vi "Remove Digital Pattern.vi"(8 "error in (no error)":errorcluster, 10 "Page Data in":T1 {"Node Ptr" format="%.0x"}, 11 "State queue in":string[](array[string])) -> (0 "error out":errorcluster, 2 "Page Data out":T1 {"Node Ptr" format="%.0x"}, 3 "State queue out":string[](array[string]))   [LabVIEW 2013, in "Engine Simulation Toolkit System Explorer.lvlib"]
uses:
  Engine Simulation Toolkit System Explorer.lvlib
  Digital Patterns Page Data.ctl
  <vilib>/NI Veristand/Custom Device API/Custom Device Item Ref.ctl
  Digital Pattern.ctl
  Digital Pattern Base.ctl
  Digital Pattern Remove Edge.ctl
  Digital Pattern Add Pulse.ctl
  <vilib>/NI Veristand/Custom Device API/Custom Device API.lvlib
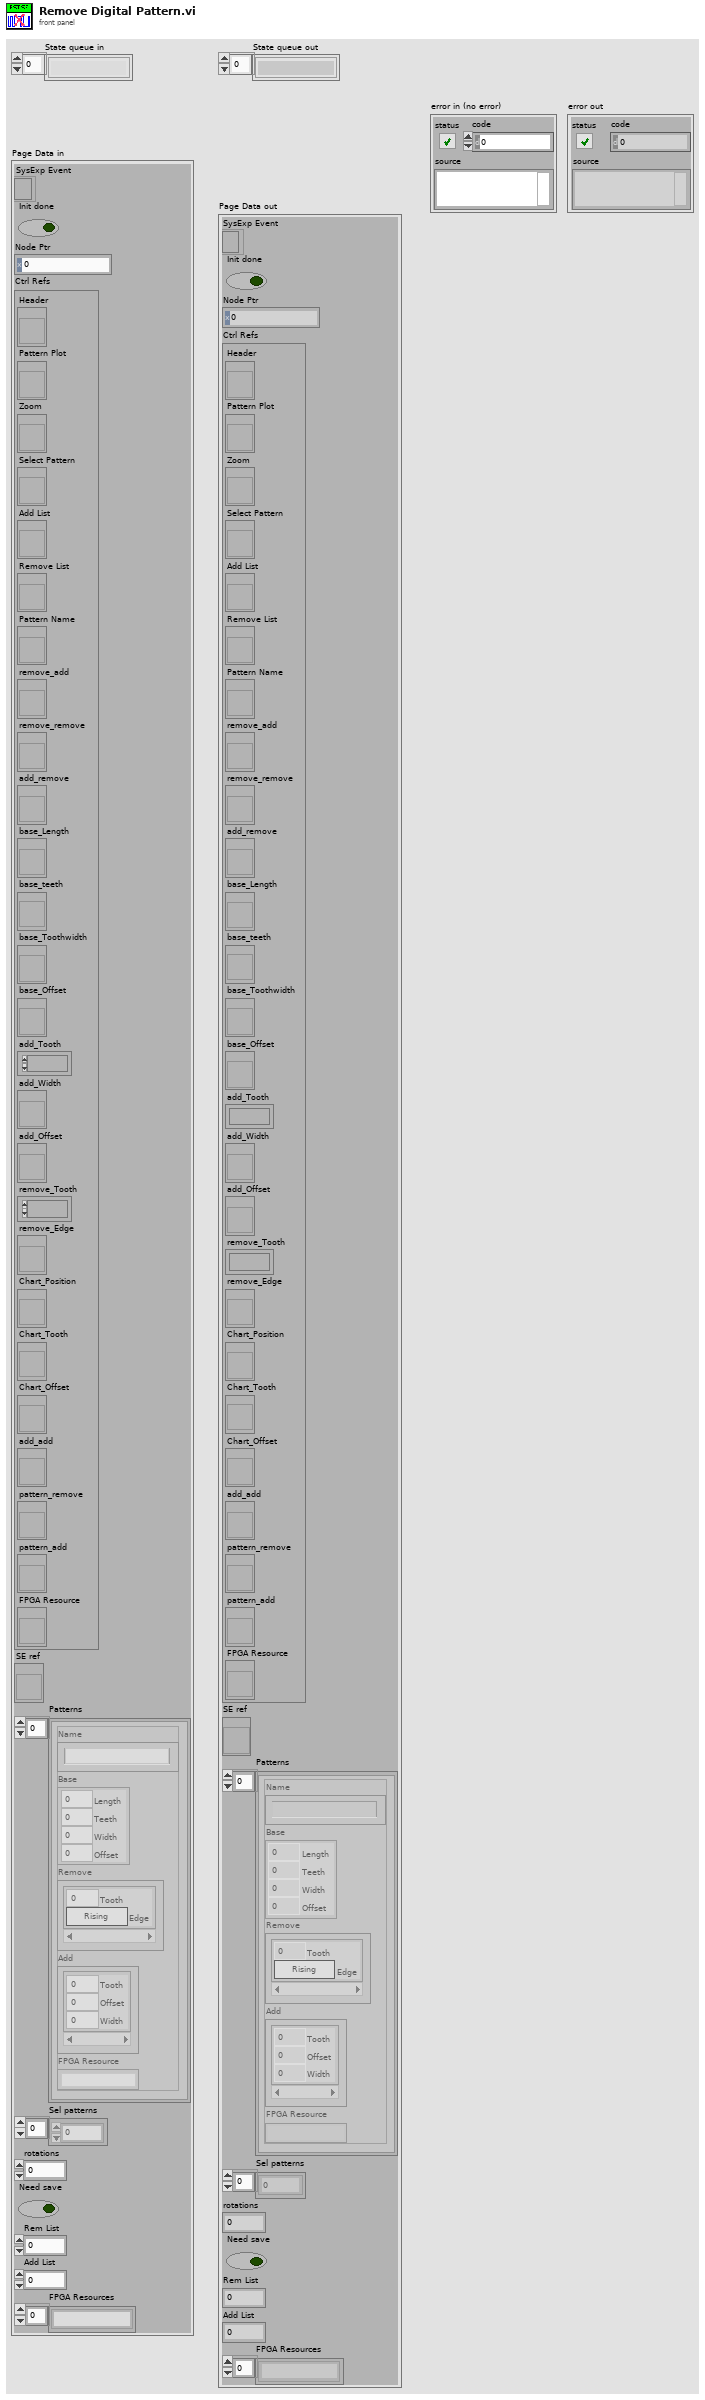
[diagram p1: front panel]
types:
  T1 = typedef "Engine Simulation Toolkit System Explorer.lvlib/Digital Patterns Page Data.ctl" = cluster{"SysExp Event":refnum<event-registration>, "Init done":bool, "Node Ptr":T2, "Ctrl Refs":cluster{"Header":refnum<vi>, "Pattern Plot":refnum<vi>, "Zoom":refnum<vi>, "Select Pattern":refnum<vi>, "Add List":refnum<vi>, "Remove List":refnum<vi>, "Pattern Name":refnum<vi>, "remove_add":refnum<vi>, "remove_remove":refnum<vi>, "add_remove":refnum<vi>, "base_Length":refnum<vi>, "base_teeth":refnum<vi>, "base_Toothwidth":refnum<vi>, "base_Offset":refnum<vi>, "add_Tooth":refnum<vi>, "add_Width":refnum<vi>, "add_Offset":refnum<vi>, "remove_Tooth":refnum<vi>, "remove_Edge":refnum<vi>, "Chart_Position":refnum<vi>, "Chart_Tooth":refnum<vi>, "Chart_Offset":refnum<vi>, "add_add":refnum<vi>, "pattern_remove":refnum<vi>, "pattern_add":refnum<vi>, "FPGA Resource":refnum<vi>}, "SE ref":refnum<vi>, "Patterns":T3[], "Sel patterns":i32[], "rotations":u16, "Need save":bool, "Rem List":i32, "Add List":i32, "FPGA Resources":string[]}
  T2 = typedef "Custom Device API.lvlib/Custom Device Item Ref.ctl" = u64
  T3 = typedef "Engine Simulation Toolkit System Explorer.lvlib/Digital Pattern.ctl" = cluster{"Name":string, "Base":T4, "Remove":T5[], "Add":T6[], "FPGA Resource":string}
  T4 = typedef "Engine Simulation Toolkit System Explorer.lvlib/Digital Pattern Base.ctl" = cluster{"Length":dbl, "Teeth":u16, "Width":dbl, "Offset":dbl}
  T5 = typedef "Engine Simulation Toolkit System Explorer.lvlib/Digital Pattern Remove Edge.ctl" = cluster{"Tooth":u16, "Edge":bool}
  T6 = typedef "Engine Simulation Toolkit System Explorer.lvlib/Digital Pattern Add Pulse.ctl" = cluster{"Tooth":u16, "Offset":dbl, "Width":dbl}
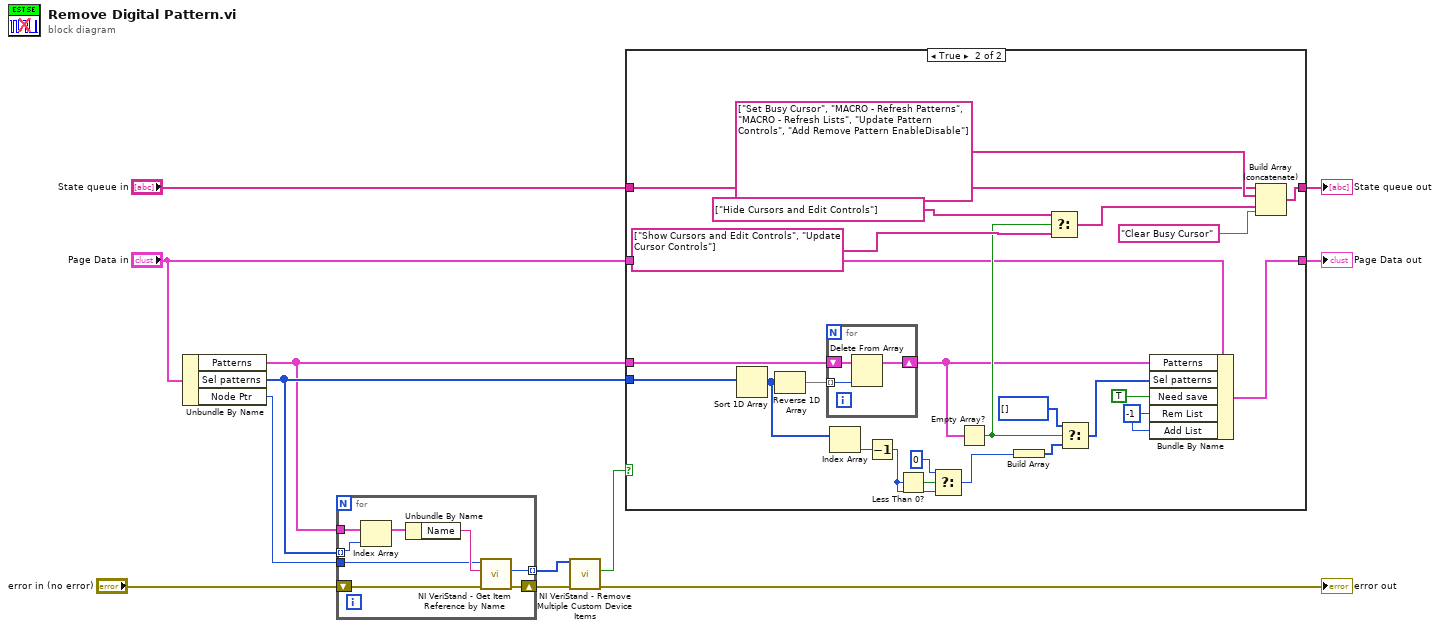
[diagram p0: block diagram]
diagram:
  n1 = Unbundle By Name("Page Data in") -> ("Patterns"=w6:T3[], "Sel patterns"=w7:i32[], "Node Ptr"=w5:T2)
  n2 = for {
    tunnel: w7 -> [w17] mode=indexing
    tunnel: w6 -> [w19]
    tunnel: w5 -> [w15]
    tunnel: [w14] -> w3 mode=indexing
    shift-right: [w13] -> w4
    shift-left: "error in (no error)" -> [w20]
    n3 = Index Array(array=w19, index=w17) -> (element=w18:T3)
    n4 = Unbundle By Name(w18) -> ("Name"=w16:string)
    n5 = call <vilib>:"NI VeriStand - Get Item Reference by Name.vi"("error in (no error)"=w20, "Item Name"=w16, "Parent Ref in"=w15) -> ("error out"=w13:errorcluster, "Item Ref"=w14:T2)  [unwired: 5 in, 2 out]
  }
  n6 = call <vilib>:"NI VeriStand - Remove Multiple Custom Device Items.vi"("error in (no error)"=w4, "Item Refs in"=w3) -> ("error out"=→"error out":errorcluster, "Deleted?"=w2:bool)  [unwired: 8 in]
  n7 = case shown="True" w2 {
    tunnel: [w22 w30] -> w12
    tunnel: [w21 w28] -> w11
    tunnel: "Page Data in" -> [w21 w27]
    tunnel: "State queue in" -> [w22 w26]
    tunnel: w7 -> [_ w24]
    tunnel: w6 -> [_ w23]
    frame False {
    }
    frame True {
      w36 = -1 ("Rem List")
      n8 = Sort 1D Array(array=w24) -> (sorted array=w37:i32[])
      n9 = Reverse 1D Array(array=w37) -> (reversed array=w25:i32[])
      n10 = for {
        tunnel: w25 -> [w50] mode=indexing
        shift-right: [w49] -> w31
        shift-left: w23 -> [w48]
        n11 = Delete From Array(array=w48, index=w50) -> (array with subset deleted=w49:T3[])  [unwired: 1 in, 1 out]
      }
      n12 = Index Array(array=w37) -> (element=w34:i32)  [unwired: 1 in]
      n13 = Decrement(x=w34) -> (x-1=w39:i32)
      n14 = Less Than 0?(x=w39) -> (x < 0?=w38:bool)
      n15 = Select(t=0, s=w38, f=w39) -> (s? t:f=w40:i32)
      n16 = Empty Array?(array=w31) -> (empty?=w43:bool)
      n17 = Build Array(w40) -> (w35:i32[])
      n18 = Select(t=string[] ["Hide Cursors and Edit Controls"], s=w43, f=string[] ["Show Cursors and Edit Controls", "Update Cursor Controls"]) -> (s? t:f=w44:string[])
      n19 = Select(t=i32[] [] ("appended array"), s=w43, f=w35) -> (s? t:f=w33:i32[])
      n20 = Bundle By Name(cluster=w27, "Patterns"=w31, "Sel patterns"=w33, "Need save"=TRUE, "Rem List"=w36, "Add List"=w36) -> (w28:T1)
      n21 = Build Array (concatenate)(w26, string[] ["Set Busy Cursor", "MACRO - Refresh Patterns", "MACRO - Refresh Lists", "Update Pattern Controls", "Add Remove Pattern EnableDisable"], w44, "Clear Busy Cursor") -> (w30:string[])
    }
  }
  "State queue out" <- w12
  "Page Data out" <- w11
